vi "pad_string.vi"(11 "string":string) -> (3 "padded_string":string)   [LabVIEW 2015, in "lv-graph.lvlib"]
uses:
  lv-graph.lvlib
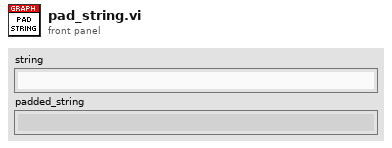
[diagram p1: front panel]
types:
  T1 = cluster{"left":i16, "top":i16, "right":i16, "bottom":i16}
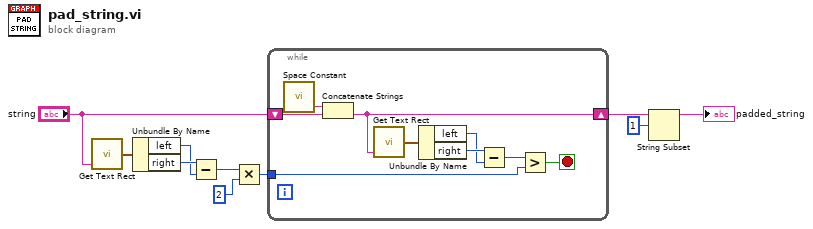
[diagram p0: block diagram]
diagram:
  n1 = call <vilib>:"Get Text Rect.vi"("text"="string") -> ("rect"=w10:T1)  [unwired: 8 in]
  n2 = Unbundle By Name(w10) -> ("left"=w8:i16, "right"=w9:i16)
  n3 = Subtract(x=w9, y=w8) -> (x-y=w6:i16)
  n4 = Multiply(x=w6, y=i16 2) -> (x*y=w4:i16)
  n5 = while {
    shift-right: [w13] -> w2
    shift-left: "string" -> [w19]
    tunnel: w4 -> [w14]
    stop <- w15 stop-if-true
    n6 = call <vilib>:"Space Constant.vi"() -> ("String"=w11:string)
    n7 = Concatenate Strings(w11, w19) -> (w13:string)
    n8 = call <vilib>:"Get Text Rect.vi"("text"=w13) -> ("rect"=w17:T1)  [unwired: 8 in]
    n9 = Unbundle By Name(w17) -> ("left"=w16:i16, "right"=w18:i16)
    n10 = Subtract(x=w18, y=w16) -> (x-y=w12:i16)
    n11 = Greater?(x=w12, y=w14) -> (0:w15:bool)
  }
  n12 = String Subset(string=w2, offset (0)=1) -> (substring=→"padded_string":string)  [unwired: 1 in]
